vi "Digital Output DAQ Engine.vi"(8 "error in":errorcluster, 10 "DAQ Engine":refnum<notifier>, 11 "Sequence Context In":refnum<k7>) -> (0 "error out":errorcluster)   [LabVIEW 2023, in "LTT_TeststandSteptypes.lvlib"]
uses:
  LTT_TeststandSteptypes.lvlib
  HardwareAbstractionLayer_LVOOP/Main/Class Ref.ctl
  HardwareAbstractionLayer_LVOOP/DMM/DMM.lvclass
  HardwareAbstractionLayer_LVOOP/Function Generator/Function Generator.lvclass
  HardwareAbstractionLayer_LVOOP/Oscilloscope/Oscilloscope.lvclass
  HardwareAbstractionLayer_LVOOP/PowerSupply/PowerSupply.lvclass
  HardwareAbstractionLayer_LVOOP/Teststand/Teststand.lvclass
  HardwareAbstractionLayer_LVOOP/Analog Output/AO/AO.lvclass
  HardwareAbstractionLayer_LVOOP/Analog Input/AI/AI.lvclass
  HardwareAbstractionLayer_LVOOP/Database/Database.lvclass
  HardwareAbstractionLayer_LVOOP/Digital Output/DO_class/DO.lvclass
  HardwareAbstractionLayer_LVOOP/Digital Input/DI_class/DI.lvclass
  HardwareAbstractionLayer_LVOOP/PWM Output/PWM Output_class/PWM Output.lvclass
  HardwareAbstractionLayer_LVOOP/PWM Input/PWM Input_class/PWM Input.lvclass
  HardwareAbstractionLayer_LVOOP/NI Switch/NISwitch_class/NISwitch.lvclass
  HardwareAbstractionLayer_LVOOP/Modbus/Modbus_class/Modbus.lvclass
  HardwareAbstractionLayer_LVOOP/CAN/CAN Lib/CAN_class/CAN.lvclass
  HardwareAbstractionLayer_LVOOP/Digital Output/NI Digital Output_class/NI Digital Output.lvclass
  D:/eDCU LTT/VT LTT Project/Source Code/HardwareAbstractionLayer_LVOOP/Digital Output/DO_class/DO.lvclass
  HardwareAbstractionLayer_LVOOP/Main/Class Options.ctl
  <vilib>/Utility/error.llb/DialogType.ctl
  HardwareAbstractionLayer_LVOOP/Main/Main.lvclass
panel:
  in  "stop":bool
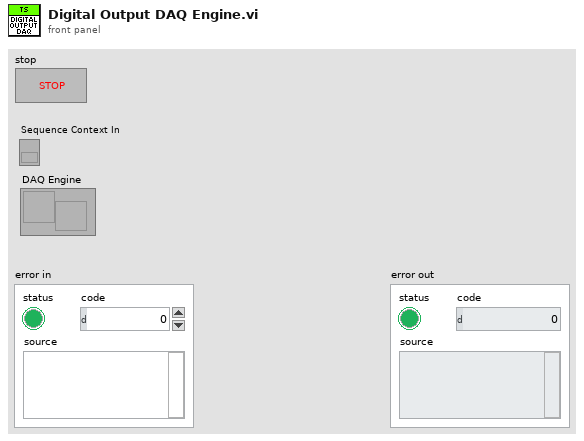
[diagram p1: front panel]
types:
  T1 = typedef "HardwareAbstractionLayer_LVOOP.lvlib/Main.lvclass/Class Ref.ctl" = cluster{"DMM":refnum<class "DMM.lvclass">, "Function Generator":refnum<class "Function Generator.lvclass">, "Oscilloscope":refnum<class "Oscilloscope.lvclass">, "PowerSupply":refnum<class "PowerSupply.lvclass">, "Teststand":refnum<class "Teststand.lvclass">, "AO":refnum<class "AO.lvclass">, "AI":refnum<class "AI.lvclass">, "Database":refnum<class "Database.lvclass">, "AO Waveform Generation":refnum<class "AO.lvclass">, "DO":refnum<class "DO.lvclass">, "DI":refnum<class "DI.lvclass">, "PWM Output":refnum<class "PWM Output.lvclass">, "PWM Input":refnum<class "PWM Input.lvclass">, "RelayOutput":refnum<class "NISwitch.lvclass">, "Modbus":refnum<class "Modbus.lvclass">, "CAN":refnum<class "CAN.lvclass">}
  T2 = typedef "HardwareAbstractionLayer_LVOOP.lvlib/Main.lvclass/Class Options.ctl" = enum16{"Init All Class", "Read All Class", "Write AI Class", "Write AO Class", "Write AO Waveform Generation", "Write DI Class", "Write DO Class", "Write PWM Input Class", "Write PWM Output Class", "Exit"}
  T3 = typedef "DialogType.ctl" = u16
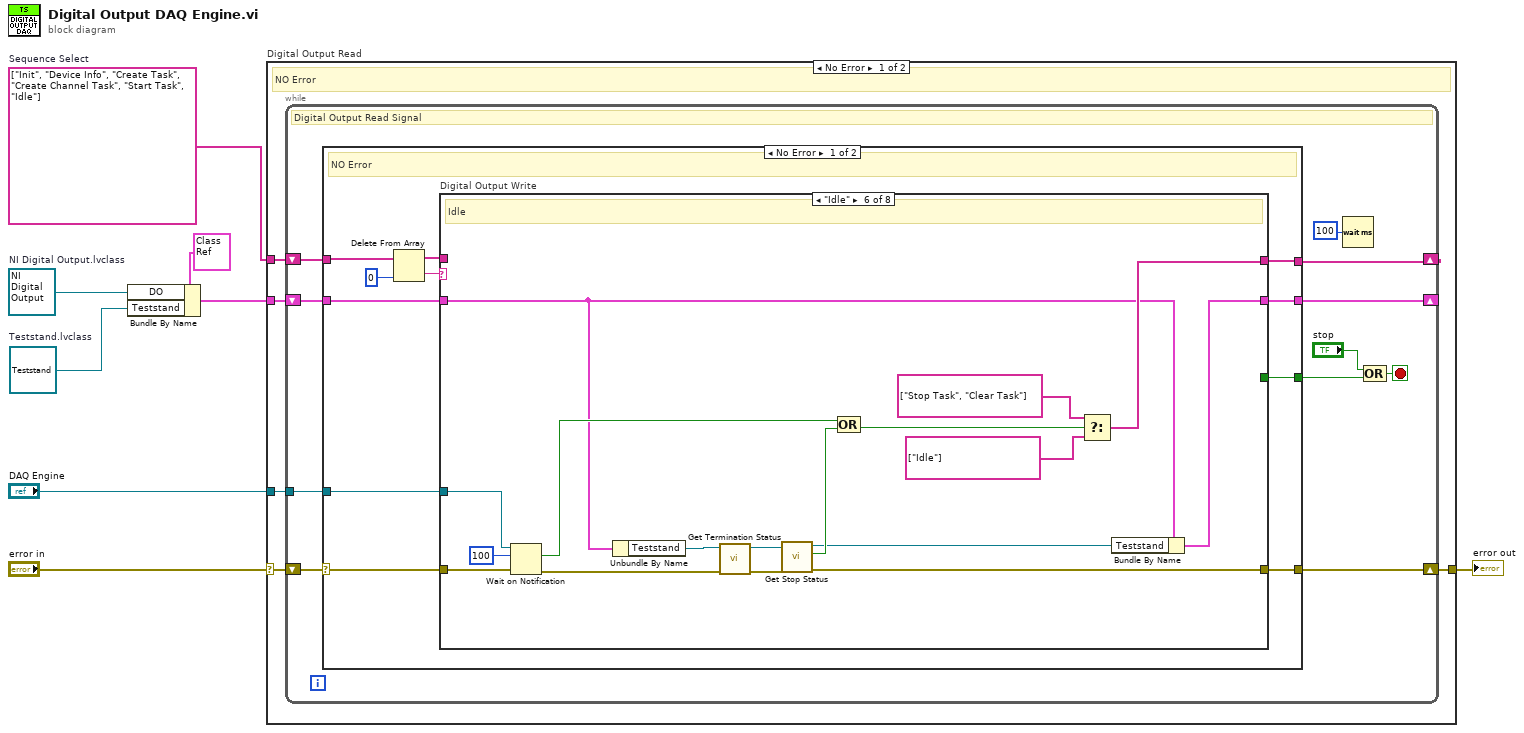
[diagram p0: block diagram]
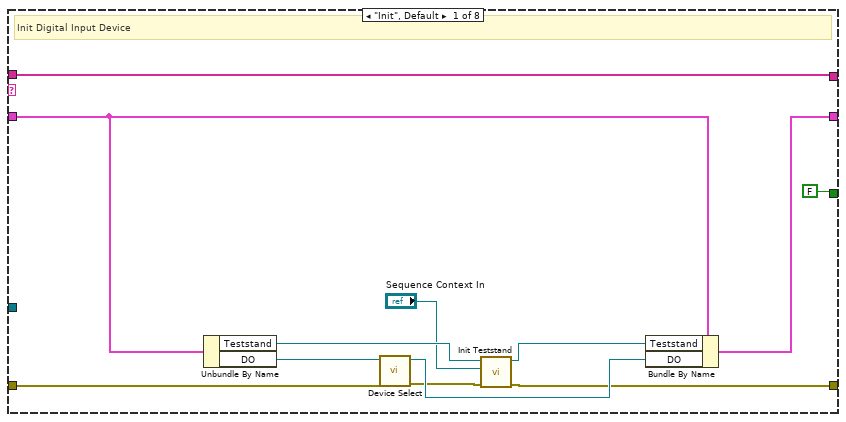
[diagram p2: hidden frame]
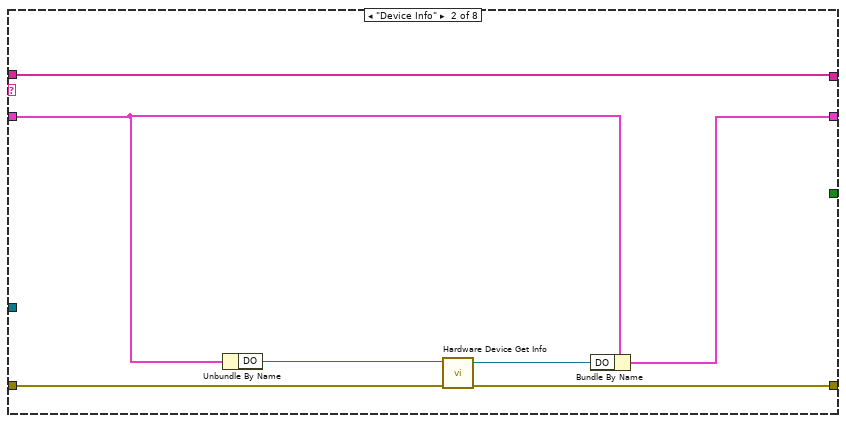
[diagram p3: hidden frame]
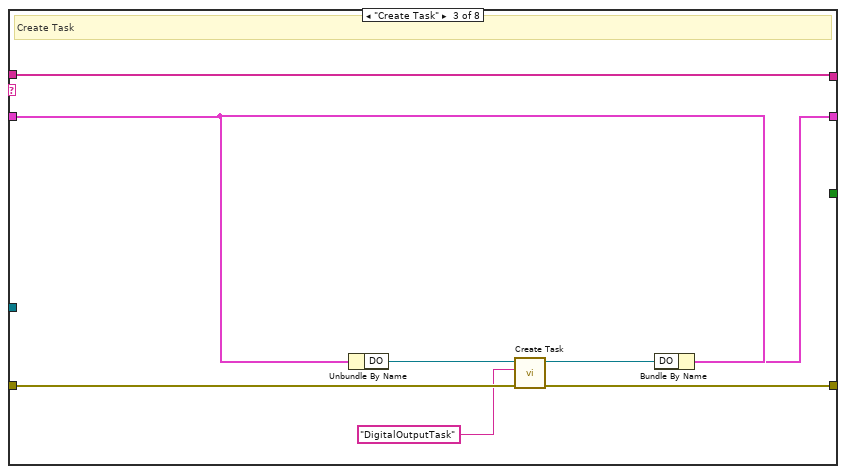
[diagram p4: hidden frame]
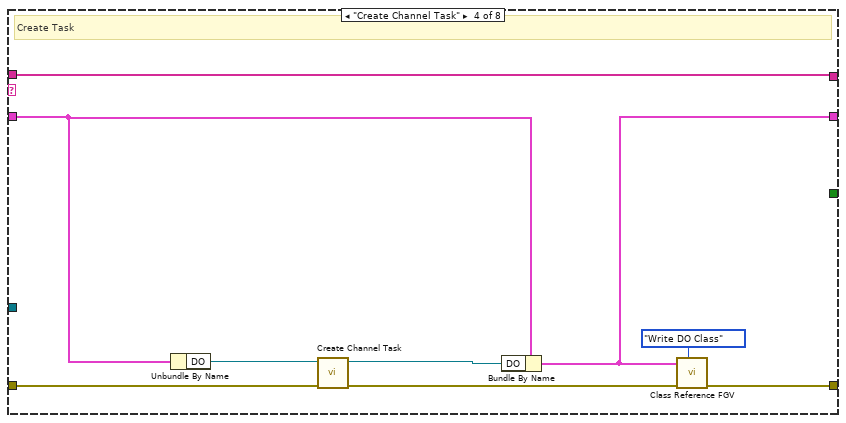
[diagram p5: hidden frame]
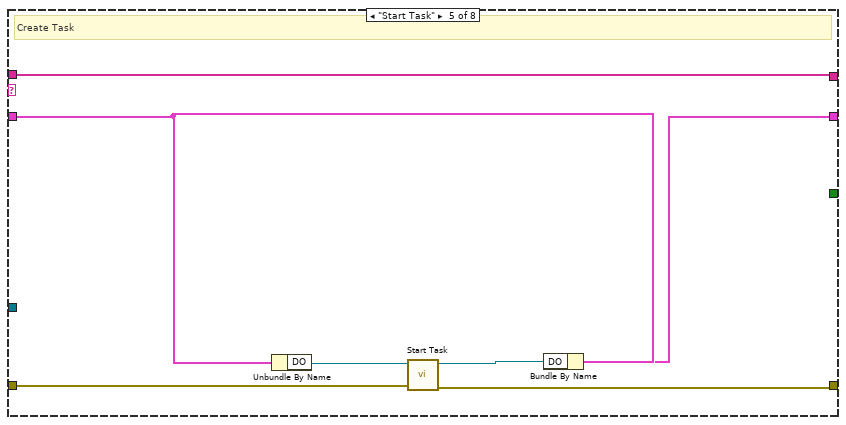
[diagram p6: hidden frame]
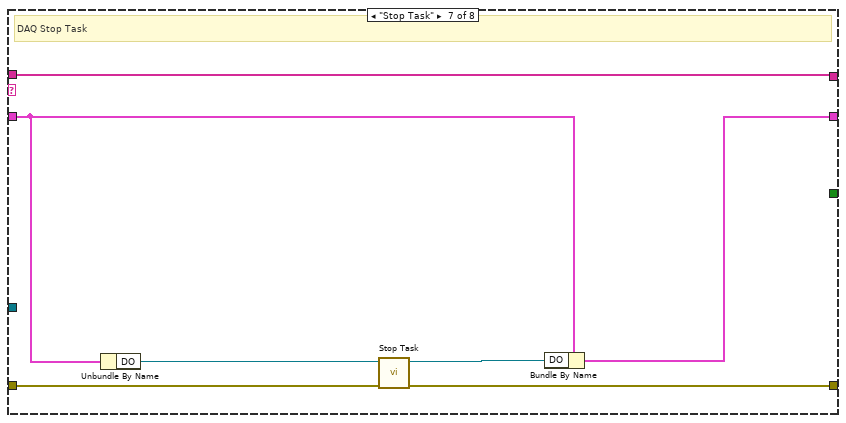
[diagram p7: hidden frame]
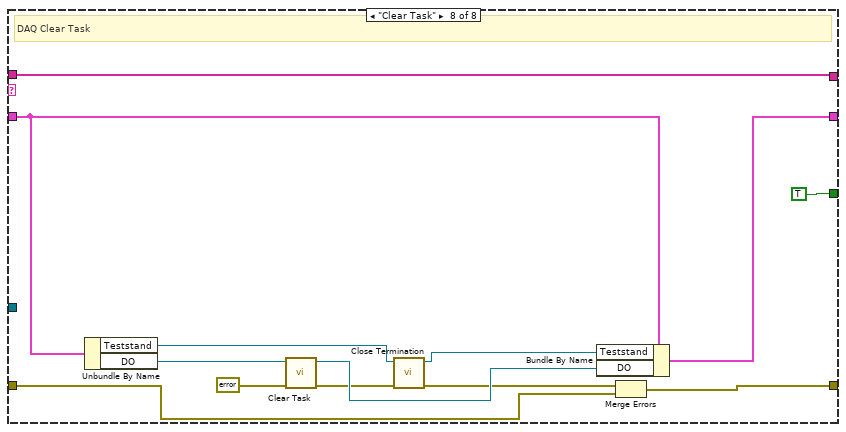
[diagram p8: hidden frame]
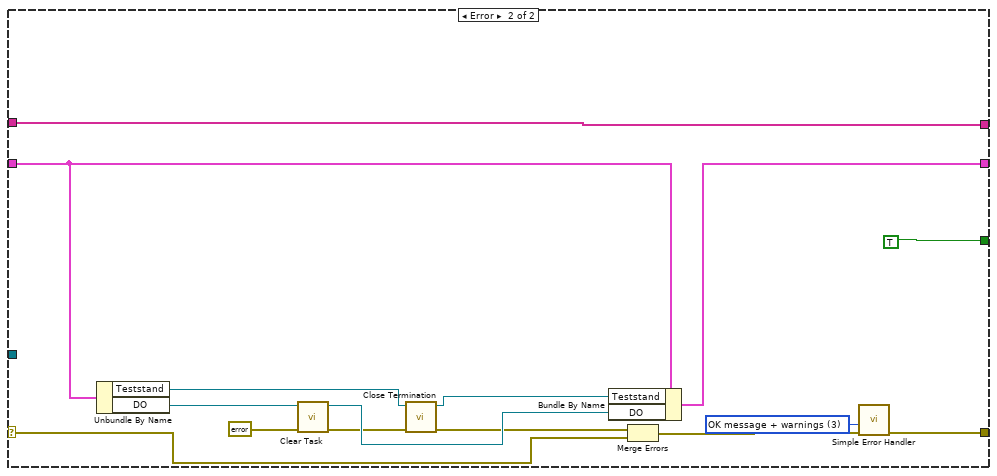
[diagram p9: hidden frame]
diagram:
  w1 = refnum<class "Teststand.lvclass"> refnum  # Teststand.lvclass
  w2 = refnum<class "NI Digital Output.lvclass"> refnum  # NI Digital Output.lvclass
  w4 = string[] ["Init", "Device Info", "Create Task", "Create Channel Task", "Start Task", "Idle"]  # Sequence Select
  n1 = Bundle By Name(cluster=T1 {"DMM"=refnum, "Function Generator"=refnum, "Oscilloscope"=refnum, "PowerSupply"=refnum, "Teststand"=refnum, "AO"=refnum, "AI"=refnum, "Database"=refnum, "AO Waveform Generation"=refnum, "DO"=refnum, "DI"=refnum, "PWM Output"=refnum, "PWM Input"=refnum, "RelayOutput"=refnum, "Modbus"=refnum, "CAN"=refnum} ("Class Cluster"), "DO"=w2, "Teststand"=w1) -> (w5:T1)
  n2 = case "Digital Output Read" shown="No Error" "error in" {
    selector: "error in" -> [w13 w131]
    tunnel: [w12 w131] -> w7
    tunnel: w5 -> [w11 _]
    tunnel: w4 -> [w10 _]
    tunnel: "DAQ Engine" -> [w9 _]
    frame No Error {
      # "NO Error"
      n3 = while {
        shift-right: [w23] -> w12
        shift-left: w13 -> [w24]
        shift-right: [w21] -> _
        shift-left: w11 -> [w22]
        shift-right: [w19] -> _
        shift-left: w10 -> [w20]
        tunnel: w9 -> [w14]
        stop <- w16 stop-if-true
        # "Digital Output Read Signal"
        n4 = case shown="No Error" w24 {
          selector: w24 -> [w35 w122]
          tunnel: [w34 w117] -> w23
          tunnel: w22 -> [w30 w119]
          tunnel: [w29 w118] -> w21
          tunnel: w20 -> [w33 w120]
          tunnel: [w27 w120] -> w19
          tunnel: [w26 TRUE] -> w15
          tunnel: w14 -> [w25 _]
          frame No Error {
            # "NO Error"
            n5 = Delete From Array(array=w33, index=0) -> (deleted portion=w32:string, array with subset deleted=w28:string[])  [unwired: 1 in]
            n6 = case "Digital Output Write" shown="\"Idle\"" w32 {
              tunnel: w35 -> [w43 w51 w59 w69 w75 w95 w99 w108]
              tunnel: [w36 w50 w58 w65 w73 w83 w98 w109] -> w34
              tunnel: w30 -> [w46 w53 w61 w70 w77 w81 w101 w114]
              tunnel: [w45 w52 w60 w63 w76 w79 w100 w113] -> w29
              tunnel: w28 -> [w47 w54 w62 w71 w78 _ w102 w115]
              tunnel: [w47 w54 w62 w71 w78 w92 w102 w115] -> w27
              tunnel: [FALSE _ _ _ _ _ _ TRUE] -> w26
              tunnel: w25 -> [_ _ _ _ _ w90 _ _]
              frame "Init", Default {
                # "Init Digital Input Device"
                n7 = Unbundle By Name(w46) -> ("Teststand"=w40:refnum<class "Teststand.lvclass">, "DO"=w42:refnum<class "DO.lvclass">)
                n8 = call-dynamic "Device Select.vi"("error in (no error)"=w43, "DO in"=w42) -> ("error out"=w37:errorcluster, "DO out"=w41:refnum<class "DO.lvclass">)  [unwired: 8 in]
                n9 = call-dynamic "Init Teststand.vi"("error in (no error)"=w37, "Sequence Context In"="Sequence Context In", "Teststand in"=w40) -> ("error out"=w36:errorcluster, "Teststand out"=w39:refnum<class "Teststand.lvclass">)  [unwired: 7 in]
                n10 = Bundle By Name(cluster=w46, "Teststand"=w39, "DO"=w41) -> (w45:T1)
              }
              frame "Device Info" {
                n11 = Unbundle By Name(w53) -> ("DO"=w48:refnum<class "DO.lvclass">)
                n12 = call-dynamic "Hardware Device Get Info.vi"("error in (no error)"=w51, "DO in"=w48) -> ("error out"=w50:errorcluster, "DO out"=w49:refnum<class "DO.lvclass">)  [unwired: 8 in]
                n13 = Bundle By Name(cluster=w53, "DO"=w49) -> (w52:T1)
              }
              frame "Create Task" {
                # "Create Task"
                n14 = Unbundle By Name(w61) -> ("DO"=w56:refnum<class "DO.lvclass">)
                n15 = call-dynamic "Create Task.vi"("error in (no error)"=w59, "Task Name"="DigitalOutputTask", "DO in"=w56) -> ("error out"=w58:errorcluster, "DO out"=w57:refnum<class "DO.lvclass">)  [unwired: 7 in]
                n16 = Bundle By Name(cluster=w61, "DO"=w57) -> (w60:T1)
              }
              frame "Create Channel Task" {
                # "Create Task"
                n17 = Unbundle By Name(w70) -> ("DO"=w67:refnum<class "DO.lvclass">)
                n18 = call-dynamic "Create Channel Task.vi"("error in (no error)"=w69, "DO in"=w67) -> ("error out"=w66:errorcluster, "DO out"=w68:refnum<class "DO.lvclass">)  [unwired: 8 in]
                n19 = Bundle By Name(cluster=w70, "DO"=w68) -> (w63:T1)
                n20 = call "Class Reference FGV.vi"("Options"=Class_Options."Write DO Class", "error in"=w66, "Class Cluster In"=w63) -> ("error out"=w65:errorcluster)  [unwired: 7 in, 1 out]
              }
              frame "Start Task" {
                # "Create Task"
                n21 = Unbundle By Name(w77) -> ("DO"=w74:refnum<class "DO.lvclass">)
                n22 = call-dynamic "Start Task.vi"("error in (no error)"=w75, "DO in"=w74) -> ("error out"=w73:errorcluster, "DO out"=w72:refnum<class "DO.lvclass">)  [unwired: 8 in]
                n23 = Bundle By Name(cluster=w77, "DO"=w72) -> (w76:T1)
              }
              frame "Idle" {
                # "Idle"
                n24 = Wait on Notification(notifier=w90, timeout in ms (-1)=100, error in (no error)=w95) -> (notification=w88:bool, error out=w84:errorcluster)  [unwired: 1 in, 2 out]
                n25 = Unbundle By Name(w81) -> ("Teststand"=w87:refnum<class "Teststand.lvclass">)
                n26 = call-dynamic "Get Termination Status.vi"("error in (no error)"=w84, "Teststand in"=w87) -> ("error out"=w86:errorcluster, "Teststand out"=w85:refnum<class "Teststand.lvclass">)  [unwired: 7 in, 1 out]
                n27 = call-dynamic "Get Stop Status.vi"("error in (no error)"=w86, "Teststand in"=w85) -> ("error out"=w83:errorcluster, "Value"=w82:bool, "Teststand out"=w80:refnum<class "Teststand.lvclass">)  [unwired: 7 in]
                n28 = Compound Arithmetic op=OR(w88, w82) -> (w91:bool)
                n29 = Select(t=string[] ["Stop Task", "Clear Task"], s=w91, f=string[] ["Idle"]) -> (s? t:f=w92:string[])
                n30 = Bundle By Name(cluster=w81, "Teststand"=w80) -> (w79:T1)
              }
              frame "Stop Task" {
                # "DAQ Stop Task"
                n31 = Unbundle By Name(w101) -> ("DO"=w96:refnum<class "DO.lvclass">)
                n32 = call-dynamic "Stop Task.vi"("error in (no error)"=w99, "DO in"=w96) -> ("error out"=w98:errorcluster, "DO out"=w97:refnum<class "DO.lvclass">)  [unwired: 8 in]
                n33 = Bundle By Name(cluster=w101, "DO"=w97) -> (w100:T1)
              }
              frame "Clear Task" {
                # "DAQ Clear Task"
                n34 = Unbundle By Name(w114) -> ("Teststand"=w106:refnum<class "Teststand.lvclass">, "DO"=w111:refnum<class "DO.lvclass">)
                n35 = call-dynamic "Clear Task.vi"("error in (no error)"=errorcluster {"status"=FALSE, "code"=0, "source"=""}, "DO in"=w111) -> ("error out"=w105:errorcluster, "DO out"=w110:refnum<class "DO.lvclass">)  [unwired: 8 in]
                n36 = call-dynamic "Close Termination.vi"("error in (no error)"=w105, "Teststand in"=w106) -> ("error out"=w104:errorcluster, "Teststand out"=w103:refnum<class "Teststand.lvclass">)  [unwired: 8 in]
                n37 = Bundle By Name(cluster=w114, "Teststand"=w103, "DO"=w110) -> (w113:T1)
                n38 = Merge Errors(w104, w108) -> (w109:errorcluster)
              }
            }
          }
          frame Error {
            w116 = T3 3 items=["no dialog", "OK message", "continue or stop message", "OK message + warnings", "continue/stop + warnings"] ("type of dialog (OK msg:1)")
            n39 = Unbundle By Name(w119) -> ("Teststand"=w126:refnum<class "Teststand.lvclass">, "DO"=w129:refnum<class "DO.lvclass">)
            n40 = call-dynamic "Clear Task.vi"("error in (no error)"=errorcluster {"status"=FALSE, "code"=0, "source"=""}, "DO in"=w129) -> ("error out"=w125:errorcluster, "DO out"=w128:refnum<class "DO.lvclass">)  [unwired: 8 in]
            n41 = call-dynamic "Close Termination.vi"("error in (no error)"=w125, "Teststand in"=w126) -> ("error out"=w124:errorcluster, "Teststand out"=w123:refnum<class "Teststand.lvclass">)  [unwired: 8 in]
            n42 = Bundle By Name(cluster=w119, "Teststand"=w123, "DO"=w128) -> (w118:T1)
            n43 = Merge Errors(w124, w122) -> (w121:errorcluster)
            n44 = call <vilib>:"Simple Error Handler.vi"("type of dialog (OK msg:1)"=w116, "error in (no error)"=w121) -> ("error out"=w117:errorcluster)  [unwired: 3 in, 4 out]
          }
        }
        n45 = Wait (ms)(milliseconds to wait=u32 100) -> ()  [unwired: 1 out]
        n46 = Compound Arithmetic op=OR("stop", w15) -> (w16:bool)
      }
    }
    frame Error {
      # "Error"
    }
  }
  "error out" <- w7
